vi "Set Transfer Groups.vi"(10 "Transfer Groups":refnum<class "Transfer Group.lvclass">[](array[class]), 11 "Transceiver Thread in":refnum<class "Plugin Thread.lvclass">) -> (3 "Transceiver Thread out":refnum<class "Plugin Thread.lvclass">)   [LabVIEW 2017, in "DSF Core.lvlib" / "Plugin Thread.lvclass"]
uses:
  Thread/Plugin/Plugin Thread.lvclass
  Transfer Group/Transfer Group.lvclass
  Thread/Plugin/Plugin Thread.lvclass/Plugin Thread.ctl
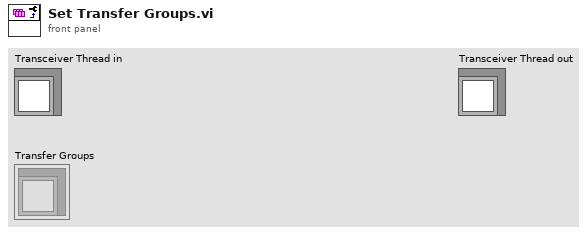
[diagram p1: front panel]
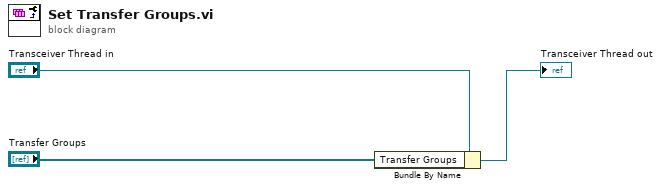
[diagram p0: block diagram]
diagram:
  n1 = Bundle By Name(cluster="Transceiver Thread in", "Transfer Groups"="Transfer Groups") -> (→"Transceiver Thread out":refnum<class "Plugin Thread.lvclass">)
